vi "Set Data Bus Tristate.vi"(8 "error in (no error)":errorcluster, 10 "Tristate":bool=TRUE, 11 "IO in":refnum<class "IO.lvclass">) -> (0 "error out":errorcluster, 3 "IO out":refnum<class "IO.lvclass">)   [LabVIEW 2021, in "IO.lvclass"]
uses:
  IO.lvclass
  IO.lvclass/IO.ctl
  <resource>/objmgr/daqmx.rc
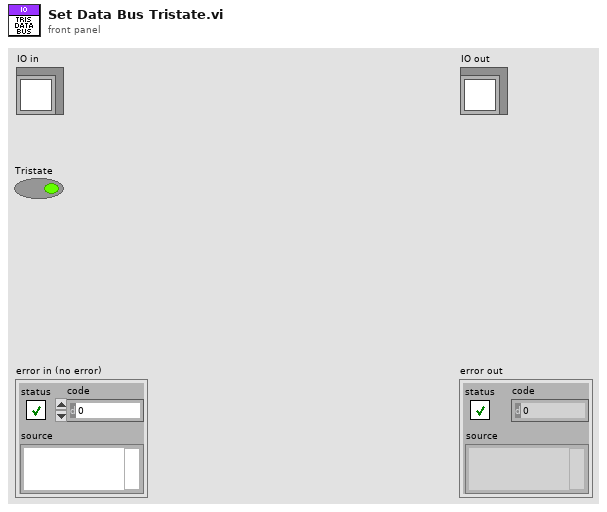
[diagram p1: front panel]
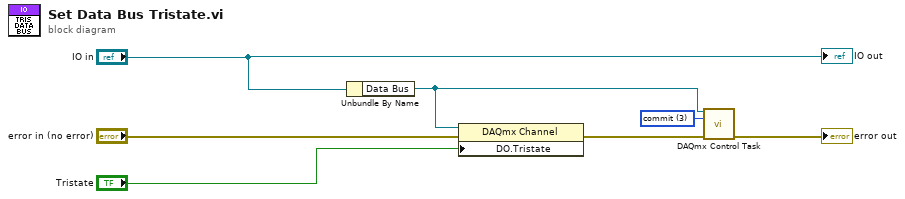
[diagram p0: block diagram]
diagram:
  w4 = 3 items=["verify"=2, "reserve"=4, "commit"=3, "unreserve"=5, "abort"=6] ("action")
  n1 = Unbundle By Name("IO in") -> ("Data Bus"=w3:refnum<k21>)
  n2 = property class="DAQmx Channel"(reference=w3, error in="error in (no error)", "DO.Tristate"="Tristate") -> (error out=w2:errorcluster)  [unwired: 1 out]
  n3 = call <vilib>:"DAQmx Control Task.vi"("task/channels in"=w3, "action"=w4, "error in"=w2) -> ("error out"=→"error out":errorcluster)  [unwired: 11 in, 1 out]
  "IO out" <- "IO in"
